vi "Ej_15_PWM_DAQ.vi"() -> ()   [LabVIEW 2021]
panel:
  in  "Amplitud":dbl=1.7 caption="Offset"
  out "Waveform Graph":dynamicdata(graph)
  in  "stop":bool
  in  "Duty Cycle (%)":dbl=5.0
  in  "Frequency":dbl=50.0
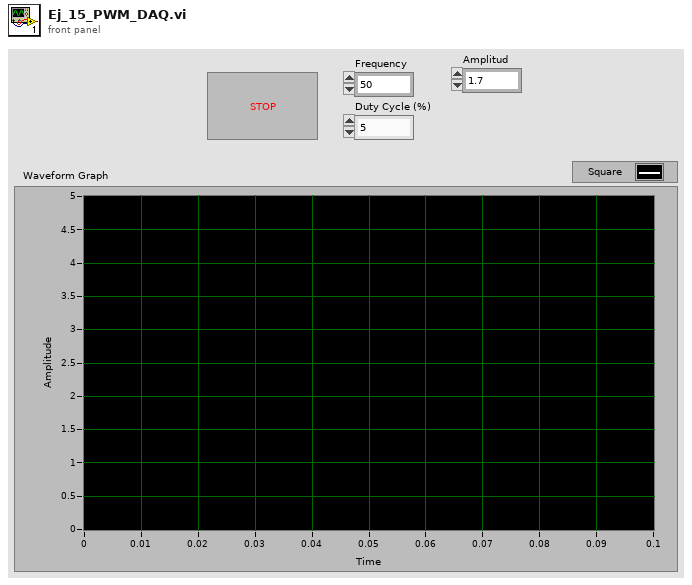
[diagram p1: front panel]
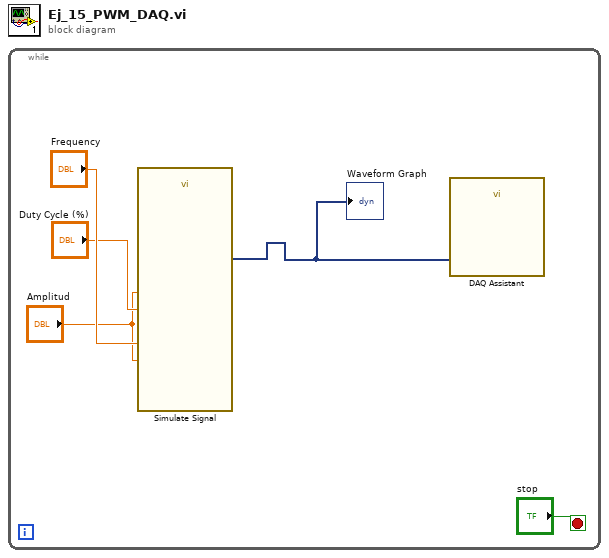
[diagram p0: block diagram]
diagram:
  n1 = while {
    stop <- "stop" stop-if-true
    n2 = call "Simulate Signal"("Offset"="Amplitud", "Duty Cycle (%)"="Duty Cycle (%)", "Frequency"="Frequency", "Amplitude"="Amplitud") -> ("Square"=w2:dynamicdata)  [unwired: 10 in, 1 out]
    "Waveform Graph" <- w2
    n3 = call "DAQ Assistant"("data"=w2) -> ()  [unwired: 17 in, 2 out]
  }
